vi "Teleop.vi"(10 "Match Info":T1={"Autonomous Elapsed Seconds"=0.0, "TeleOp Elapsed Seconds"=0.0, "Disabled Elapsed Seconds"=0.0, "Visited Autonomous"=FALSE, "Visited TeleOp"=FALSE, "Visited Disabled"=FALSE, "Autonomous Settings"={"Autonomous Style"=enum."Independent", "VI Refnum"=refnum}}, 11 "Call Context":T2) -> ()   [LabVIEW 2018]
doc: "This VI is called for each enabled TeleOp packet received from the DS. It is typically used to read from joysticks and other inputs and update I/O or setpoints for timed control loops. It should complete and return within 20 milliseconds or risk missing DS packets."
uses:
  <vilib>/Rock Robotics/WPI/DriverStation/WPI_DriverStationDerivedRobotMode.ctl
  <vilib>/Rock Robotics/WPI/DriverStation/WPI_DriverStationMatch Info.ctl
  <vilib>/Rock Robotics/WPI/Solenoid/WPI_SolenoidValue.ctl
  Framework/Robot Global Data.vi
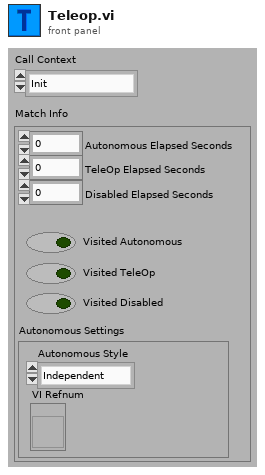
[diagram p1: front panel]
types:
  T1 = typedef "WPI_DriverStationMatch Info.ctl" = cluster{"Autonomous Elapsed Seconds":dbl, "TeleOp Elapsed Seconds":dbl, "Disabled Elapsed Seconds":dbl, "Visited Autonomous":bool, "Visited TeleOp":bool, "Visited Disabled":bool, "Autonomous Settings":cluster{"Autonomous Style":enum16{"Iterative", "Independent"}, "VI Refnum":refnum<vi>}}
  T2 = typedef "WPI_DriverStationDerivedRobotMode.ctl" = enum16{"Init", "Execute", "Stop"}
  T3 = typedef "WPI_SolenoidValue.ctl" = enum16{"Off", "On", "Forward", "Reverse"}
  T4 = typedef "Command Status Info.ctl" = cluster{"Name":string, "Status":T5, "notifier out":T6}
  T5 = typedef "Completion Status.ctl" = enum16{"Successful", "Aborted", "Incomplete"}
  T6 = typedef "Completion Notifier.ctl" = refnum<notifier>
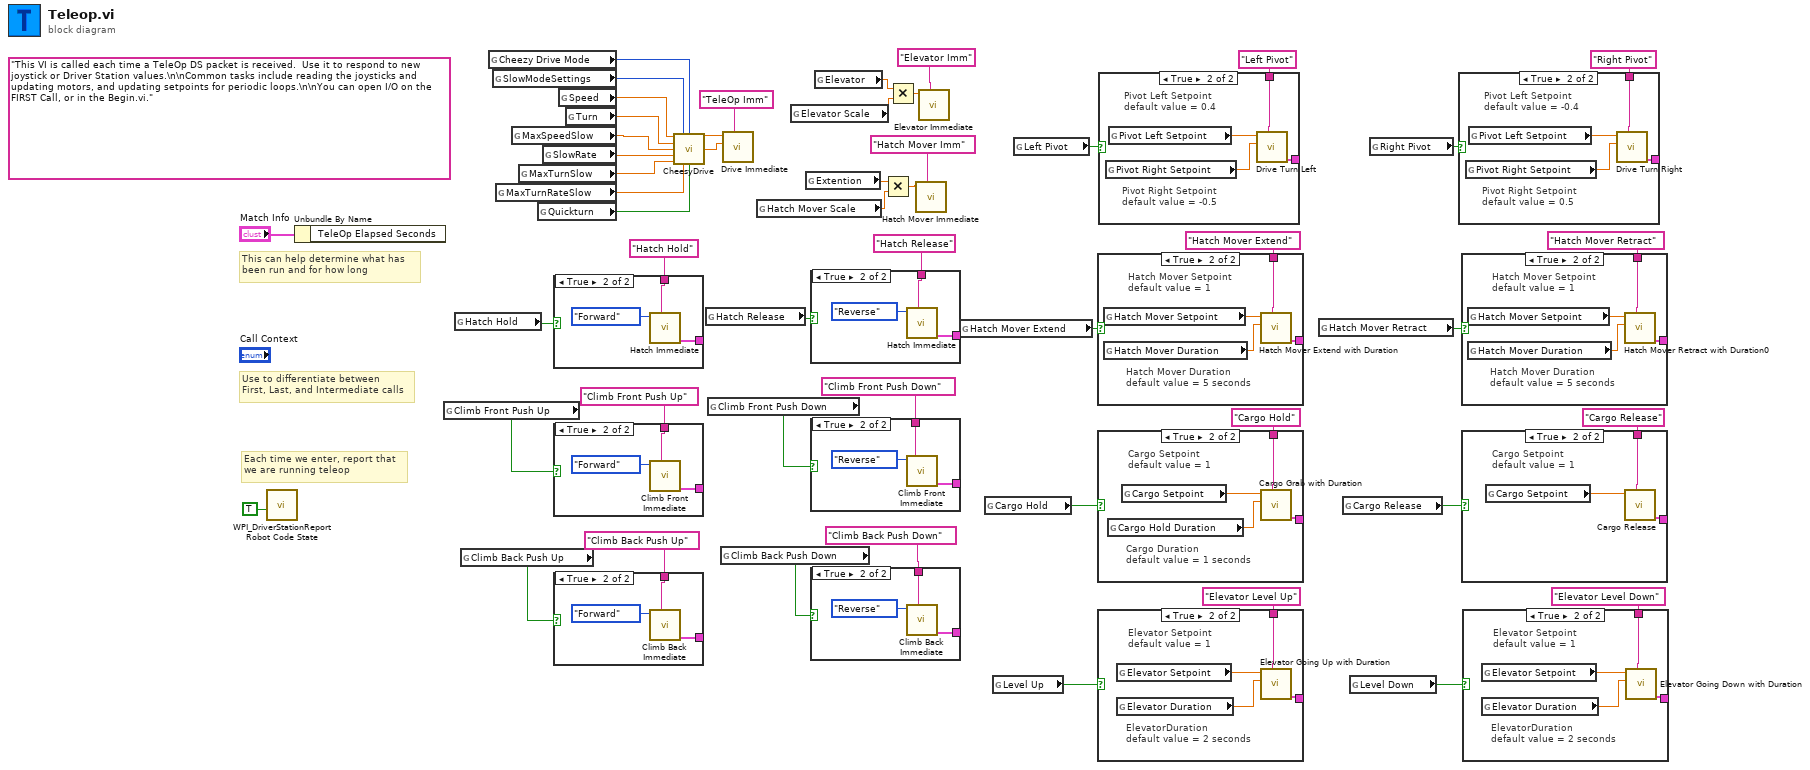
[diagram p0: block diagram]
diagram:
  (unwired) "This VI is called each time a TeleOp DS packet is received.  Use it to respond to new joystick or Driver Station values.\n\nCommon tasks include reading the joysticks and updating motors, and updating setpoints for periodic loops.\n\nYou can open I/O on the FIRST Call, or in the Begin.vi."
  # "Each time we enter, report that\nwe are running teleop"
  # "Use to differentiate between\nFirst, Last, and Intermediate calls"
  # "This can help determine what has\nbeen run and for how long"
  n1 = call <vilib>:"WPI_DriverStationReport Robot Code State.vi"("TeleOp"=TRUE ("Autonomous")) -> ()  [unwired: 10 in, 1 out]
  n2 = Unbundle By Name("Match Info") -> ()  [unwired: 1 out]
  n3 = global read "Robot Global Data.vi" "Climb Front Push Up"() -> (w42:bool)
  n4 = global read "Robot Global Data.vi" "Hatch Hold"() -> (w46:bool)
  n5 = global read "Robot Global Data.vi" "Climb Back Push Up"() -> (w39:bool)
  n6 = global read "Robot Global Data.vi" "Cheezy Drive Mode"() -> (w19:u32)
  n7 = global read "Robot Global Data.vi" "SlowModeSettings"() -> (w18:i32)
  n8 = global read "Robot Global Data.vi" "MaxTurnRateSlow"() -> (w12:dbl)
  n9 = global read "Robot Global Data.vi" "MaxSpeedSlow"() -> (w15:dbl)
  n10 = global read "Robot Global Data.vi" "MaxTurnSlow"() -> (w13:dbl)
  n11 = global read "Robot Global Data.vi" "Quickturn"() -> (w11:bool)
  n12 = global read "Robot Global Data.vi" "SlowRate"() -> (w14:dbl)
  n13 = case shown="True" w46 {
    tunnel: [_ w52] -> _
    tunnel: "Hatch Hold" ("Description") -> [_ w51]
    frame False {
    }
    frame True {
      n14 = call "Hatch Immediate.vi"("Description"=w51, "Action"=WPI_SolenoidValue."Forward") -> ("Command Info Out"=w52:T4)  [unwired: 9 in]
    }
  }
  n15 = case shown="True" w42 {
    tunnel: [_ w55] -> _
    tunnel: "Climb Front Push Up" ("Description") -> [_ w54]
    frame False {
    }
    frame True {
      n16 = call "Climb Front Immediate.vi"("Description"=w54, "Action"=WPI_SolenoidValue."Forward") -> ("Command Info Out"=w55:T4)  [unwired: 9 in]
    }
  }
  n17 = case shown="True" w39 {
    tunnel: [_ w59] -> _
    tunnel: "Climb Back Push Up" ("Description") -> [_ w58]
    frame False {
    }
    frame True {
      n18 = call "Climb Back Immediate.vi"("Description"=w58, "Relay Value"=WPI_SolenoidValue."Forward" ("Action")) -> ("Command Info Out"=w59:T4)  [unwired: 9 in]
    }
  }
  n19 = global read "Robot Global Data.vi" "Speed"() -> (w17:dbl)
  n20 = global read "Robot Global Data.vi" "Turn"() -> (w16:dbl)
  n21 = call "CheesyDrive.vi"("Throttle"=w17, "SlowModeSettings"=w18, "SlowMode"=w19, "Wheel"=w16, "MaxSpeedSlow"=w15, "SlowRate"=w14, "MaxTurnSlow"=w13, "MaxTurnRateSlow"=w12, "Quickturn"=w11) -> ("Left PWM"=w10:dbl, "Right PWM"=w9:dbl)  [unwired: 5 in]
  n22 = global read "Robot Global Data.vi" "Hatch Release"() -> (w45:bool)
  n23 = global read "Robot Global Data.vi" "Climb Front Push Down"() -> (w43:bool)
  n24 = global read "Robot Global Data.vi" "Climb Back Push Down"() -> (w38:bool)
  n25 = call "Drive Immediate.vi"("Description"="TeleOp Imm", "Right Setpoint"=w9, "Left Setpoint"=w10) -> ()  [unwired: 8 in, 1 out]
  n26 = global read "Robot Global Data.vi" "Hatch Mover Scale"() -> (w4:dbl)
  n27 = global read "Robot Global Data.vi" "Elevator Scale"() -> (w1:dbl)
  n28 = global read "Robot Global Data.vi" "Extention"() -> (w5:dbl)
  n29 = case shown="True" w45 {
    tunnel: [_ w61] -> _
    tunnel: "Hatch Release" ("Description") -> [_ w60]
    frame False {
    }
    frame True {
      n30 = call "Hatch Immediate.vi"("Description"=w60, "Action"=WPI_SolenoidValue."Reverse") -> ("Command Info Out"=w61:T4)  [unwired: 9 in]
    }
  }
  n31 = case shown="True" w43 {
    tunnel: [_ w64] -> _
    tunnel: "Climb Front Push Down" ("Description") -> [_ w63]
    frame False {
    }
    frame True {
      n32 = call "Climb Front Immediate.vi"("Description"=w63, "Action"=WPI_SolenoidValue."Reverse") -> ("Command Info Out"=w64:T4)  [unwired: 9 in]
    }
  }
  n33 = case shown="True" w38 {
    tunnel: [_ w68] -> _
    tunnel: "Climb Back Push Down" ("Description") -> [_ w67]
    frame False {
    }
    frame True {
      n34 = call "Climb Back Immediate.vi"("Description"=w67, "Relay Value"=WPI_SolenoidValue."Reverse" ("Action")) -> ("Command Info Out"=w68:T4)  [unwired: 9 in]
    }
  }
  n35 = global read "Robot Global Data.vi" "Elevator"() -> (w2:dbl)
  n36 = Multiply(x=w5, y=w4) -> (x*y=w6:dbl)
  n37 = Multiply(x=w2, y=w1) -> (x*y=w3:dbl)
  n38 = call "Hatch Mover Immediate.vi"("Description"="Hatch Mover Imm", "Setpoint"=w6) -> ()  [unwired: 9 in, 1 out]
  n39 = call "Elevator Immediate.vi"("Description"="Elevator Imm", "Setpoint"=w3) -> ()  [unwired: 9 in, 1 out]
  n40 = global read "Robot Global Data.vi" "Hatch Mover Extend"() -> (w31:bool)
  n41 = global read "Robot Global Data.vi" "Cargo Hold"() -> (w26:bool)
  n42 = global read "Robot Global Data.vi" "Level Up"() -> (w23:bool)
  n43 = global read "Robot Global Data.vi" "Left Pivot"() -> (w34:bool)
  n44 = case shown="True" w31 {
    tunnel: "Hatch Mover Extend" ("Description") -> [_ w72]
    tunnel: [_ w69] -> _
    frame False {
    }
    frame True {
      # "Hatch Mover Duration\ndefault value = 5 seconds"
      # "Hatch Mover Setpoint\ndefault value = 1"
      n45 = global read "Robot Global Data.vi" "Hatch Mover Setpoint"() -> (w71:dbl)
      n46 = global read "Robot Global Data.vi" "Hatch Mover Duration"() -> (w70:dbl)
      n47 = call "Hatch Mover Extend with Duration.vi"("Description"=w72, "Duration (s)"=w70, "Setpoint"=w71) -> ("Command Info Out"=w69:T4)  [unwired: 8 in]
    }
  }
  n48 = case shown="True" w26 {
    tunnel: "Cargo Hold" ("Description") -> [_ w76]
    tunnel: [_ w73] -> _
    frame False {
    }
    frame True {
      # "Cargo Duration\ndefault value = 1 seconds"
      # "Cargo Setpoint\ndefault value = 1"
      n49 = global read "Robot Global Data.vi" "Cargo Hold Duration"() -> (w74:dbl)
      n50 = global read "Robot Global Data.vi" "Cargo Setpoint"() -> (w75:dbl)
      n51 = call "Cargo Grab with Duration.vi"("Description"=w76, "Duration (s)"=w74, "Setpoint"=w75) -> ("Command Info Out"=w73:T4)  [unwired: 8 in]
    }
  }
  n52 = case shown="True" w23 {
    tunnel: "Elevator Level Up" ("Description") -> [_ w80]
    tunnel: [_ w77] -> _
    frame False {
    }
    frame True {
      # "ElevatorDuration\ndefault value = 2 seconds"
      # "Elevator Setpoint\ndefault value = 1"
      n53 = global read "Robot Global Data.vi" "Elevator Setpoint"() -> (w79:dbl)
      n54 = global read "Robot Global Data.vi" "Elevator Duration"() -> (w78:dbl)
      n55 = call "Elevator Going Up with Duration.vi"("Description"=w80, "Duration (s)"=w78, "Setpoint"=w79) -> ("Command Info Out"=w77:T4)  [unwired: 8 in]
    }
  }
  n56 = case shown="True" w34 {
    tunnel: "Left Pivot" ("Description") -> [_ w84]
    tunnel: [_ w81] -> _
    frame False {
    }
    frame True {
      # "Pivot Right Setpoint\ndefault value = -0.5"
      # "Pivot Left Setpoint\ndefault value = 0.4"
      n57 = global read "Robot Global Data.vi" "Pivot Right Setpoint"() -> (w82:dbl)
      n58 = global read "Robot Global Data.vi" "Pivot Left Setpoint"() -> (w83:dbl)
      n59 = call "Drive Turn Left.vi"("Description"=w84, "Right Setpoint"=w82, "Left Setpoint"=w83) -> ("Command Info Out"=w81:T4)  [unwired: 8 in]
    }
  }
  n60 = global read "Robot Global Data.vi" "Hatch Mover Retract"() -> (w28:bool)
  n61 = global read "Robot Global Data.vi" "Cargo Release"() -> (w25:bool)
  n62 = global read "Robot Global Data.vi" "Level Down"() -> (w20:bool)
  n63 = global read "Robot Global Data.vi" "Right Pivot"() -> (w33:bool)
  n64 = case shown="True" w33 {
    tunnel: "Right Pivot" ("Description") -> [_ w88]
    tunnel: [_ w85] -> _
    frame False {
    }
    frame True {
      # "Pivot Right Setpoint\ndefault value = 0.5"
      # "Pivot Left Setpoint\ndefault value = -0.4"
      n65 = global read "Robot Global Data.vi" "Pivot Right Setpoint"() -> (w86:dbl)
      n66 = global read "Robot Global Data.vi" "Pivot Left Setpoint"() -> (w87:dbl)
      n67 = call "Drive Turn Right.vi"("Description"=w88, "Right Setpoint"=w86, "Left Setpoint"=w87) -> ("Command Info Out"=w85:T4)  [unwired: 8 in]
    }
  }
  n68 = case shown="True" w28 {
    tunnel: "Hatch Mover Retract" ("Description") -> [_ w92]
    tunnel: [_ w89] -> _
    frame False {
    }
    frame True {
      # "Hatch Mover Duration\ndefault value = 5 seconds"
      # "Hatch Mover Setpoint\ndefault value = 1"
      n69 = global read "Robot Global Data.vi" "Hatch Mover Setpoint"() -> (w91:dbl)
      n70 = global read "Robot Global Data.vi" "Hatch Mover Duration"() -> (w90:dbl)
      n71 = call "Hatch Mover Retract with Duration0.vi"("Description"=w92, "Duration (s)"=w90, "Setpoint"=w91) -> ("Command Info Out"=w89:T4)  [unwired: 8 in]
    }
  }
  n72 = case shown="True" w25 {
    tunnel: "Cargo Release" ("Description") -> [_ w95]
    tunnel: [_ w93] -> _
    frame False {
    }
    frame True {
      # "Cargo Setpoint\ndefault value = 1"
      n73 = global read "Robot Global Data.vi" "Cargo Setpoint"() -> (w94:dbl)
      n74 = call "Cargo Release.vi"("Description"=w95, "Setpoint"=w94) -> ("Command Info Out"=w93:T4)  [unwired: 9 in]
    }
  }
  n75 = case shown="True" w20 {
    tunnel: "Elevator Level Down" ("Description") -> [_ w99]
    tunnel: [_ w96] -> _
    frame False {
    }
    frame True {
      # "ElevatorDuration\ndefault value = 2 seconds"
      # "Elevator Setpoint\ndefault value = 1"
      n76 = global read "Robot Global Data.vi" "Elevator Setpoint"() -> (w98:dbl)
      n77 = global read "Robot Global Data.vi" "Elevator Duration"() -> (w97:dbl)
      n78 = call "Elevator Going Down with Duration.vi"("Description"=w99, "Duration (s)"=w97, "Setpoint"=w98) -> ("Command Info Out"=w96:T4)  [unwired: 8 in]
    }
  }
